vi "Lookup Client Queue from GUID.vi"(8 "error in (no error)":errorcluster, 10 "GUID":string, 11 "Server Controller in":refnum<class "Server Controller.lvclass">) -> (0 "error out":errorcluster, 1 "found":bool, 2 "Caller-To-Actor Enqueuer":refnum<class "Message Enqueuer.lvclass">, 3 "Server Controller out":refnum<class "Server Controller.lvclass">)   [LabVIEW 2013, in "Server Controller.lvlib" / "Server Controller.lvclass"]
doc: "Returns the message queue for a client LNA based on the Connection ID"
uses:
  Server Controller.lvclass
  <vilib>/ActorFramework/Message Enqueuer/Message Enqueuer.lvclass
  Server Controller.lvclass/Server Controller.ctl
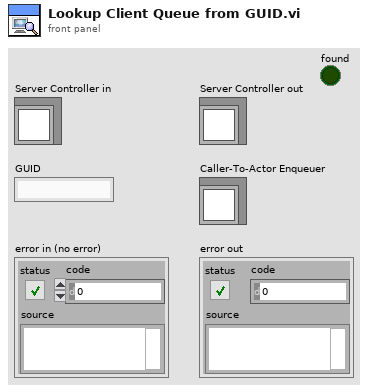
[diagram p1: front panel]
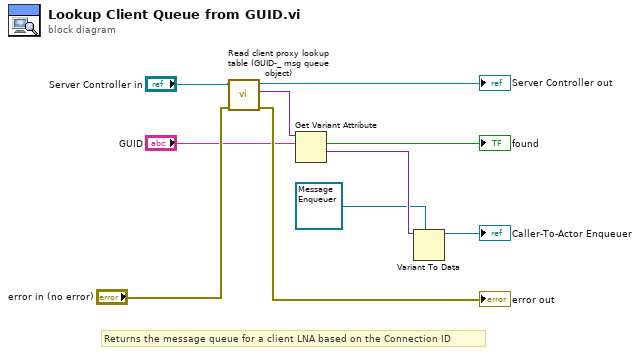
[diagram p0: block diagram]
diagram:
  # "Returns the message queue for a client LNA based on the Connection ID"
  n1 = call "Read client proxy lookup table (GUID-_ msg queue object).vi"("error in (no error)"="error in (no error)", "Server Controller in"="Server Controller in") -> ("error out"=→"error out":errorcluster, "client proxy lookup table (clientname -> msg queue object)"=w3:variant, "Server Controller out"=→"Server Controller out":refnum<class "Server Controller.lvclass">)  [unwired: 7 in]
  n2 = Get Variant Attribute(Variant=w3, name="GUID") -> (found=→"found":bool, value=w6:variant)  [unwired: 2 in, 2 out]
  n3 = Variant To Data(type=refnum<class "Message Enqueuer.lvclass"> refnum ("Caller-To-Actor Enqueuer"), Variant=w6) -> (data=→"Caller-To-Actor Enqueuer":refnum<class "Message Enqueuer.lvclass">)  [unwired: 1 in, 1 out]
